vi "ArmPassThroughBodyWristAngle.vi"(0 "Arm Pass Through Params":T2, 1 "RobotDimensions":T1, 2 "PathIn":T3[](array[typedef])) -> (6 "PathOut":T3[](array[typedef]))   [LabVIEW 2018]
uses:
  TypeDefs/ArmCoordinate.ctl
  TypeDefs/ArmPassThroughParams.ctl
  TypeDefs/ConfigComponents/Config_Dimensions.ctl
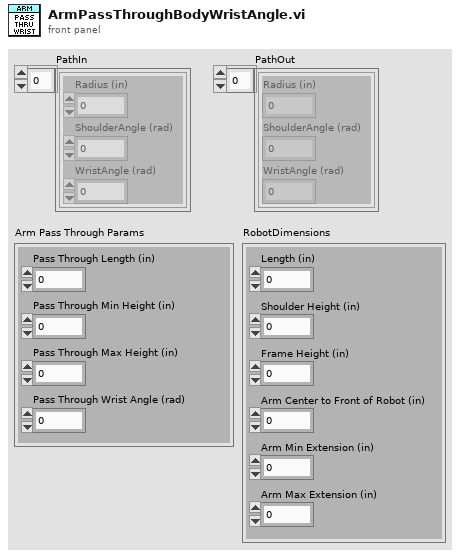
[diagram p1: front panel]
types:
  T1 = typedef "Config_Dimensions.ctl" = cluster{"Length (in)":dbl, "Shoulder Height (in)":dbl, "Frame Height (in)":dbl, "Arm Center to Front of Robot (in)":dbl, "Arm Min Extension (in)":dbl, "Arm Max Extension (in)":dbl}
  T2 = typedef "ArmPassThroughParams.ctl" = cluster{"Pass Through Length (in)":dbl, "Pass Through Min Height (in)":dbl, "Pass Through Max Height (in)":dbl, "Pass Through Wrist Angle (rad)":dbl}
  T3 = typedef "ArmCoordinate.ctl" = cluster{"Radius (in)":dbl, "ShoulderAngle (rad)":dbl, "WristAngle (rad)":dbl}
  T4 = typedef "ArmAbsolutePosition.ctl" = cluster{"X (in)":dbl, "Y (in)":dbl, "Wrist (rad)":dbl}
  T5 = typedef "ArgosLib.lvlib/Point2D.ctl" = cluster{"X (in)":dbl, "Y (in)":dbl}
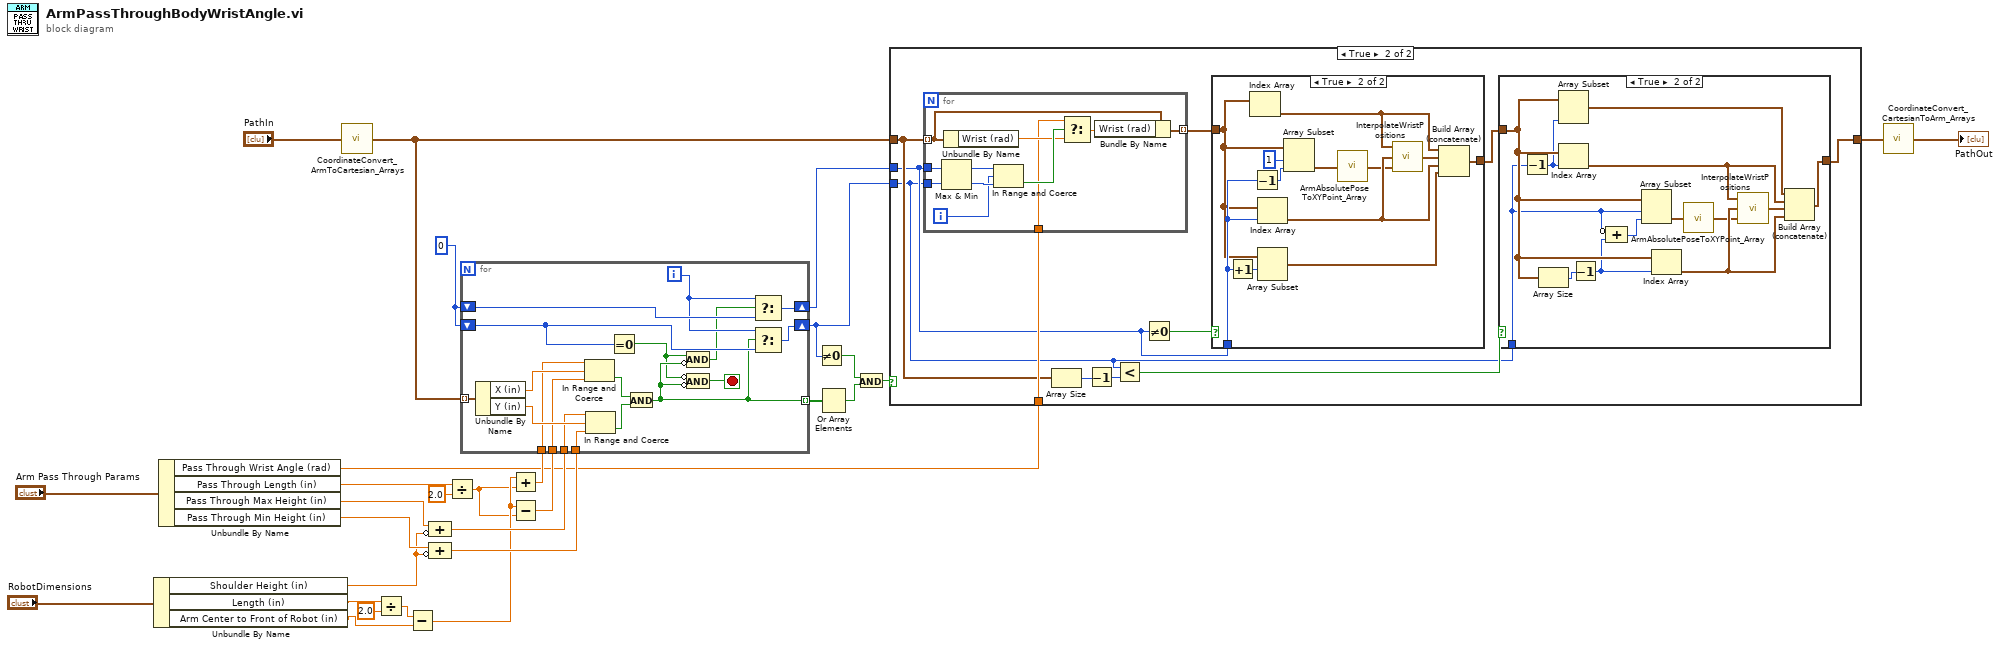
[diagram p0: block diagram]
diagram:
  w12 = 0
  n1 = Unbundle By Name("RobotDimensions") -> ("Shoulder Height (in)"=w21:dbl, "Length (in)"=w26:dbl, "Arm Center to Front of Robot (in)"=w24:dbl)
  n2 = Unbundle By Name("Arm Pass Through Params") -> ("Pass Through Wrist Angle (rad)"=w3:dbl, "Pass Through Length (in)"=w17:dbl, "Pass Through Max Height (in)"=w23:dbl, "Pass Through Min Height (in)"=w22:dbl)
  n3 = call "CoordinateConvert_ArmToCartesian_Arrays.vi"("ArmCoordinates"="PathIn") -> ("XYPoints"=w11:T4[])
  n4 = Divide(x=w26, y=2.0) -> (x/y=w25:dbl)
  n5 = Subtract(x=w25, y=w24) -> (x-y=w2:dbl)
  n6 = Compound Arithmetic op=ADD(w23, invert w21) -> (w14:dbl)
  n7 = Compound Arithmetic op=ADD(w22, invert w21) -> (w13:dbl)
  n8 = Divide(x=w17, y=2.0) -> (x/y=w1:dbl)
  n9 = Add(x=w2, y=w1) -> (x+y=w16:dbl)
  n10 = Subtract(x=w2, y=w1) -> (x-y=w15:dbl)
  n11 = for {
    tunnel: w11 -> [w47] mode=indexing
    tunnel: w16 -> [w44]
    tunnel: w15 -> [w43]
    tunnel: w14 -> [w42]
    tunnel: w13 -> [w41]
    tunnel: [w31] -> w10 mode=indexing
    shift-right: [w36] -> w4
    shift-left: w12 -> [w35]
    shift-right: [w38] -> w5
    shift-left: w12 -> [w37]
    i -> [w34]
    stop <- w32 stop-if-true
    n12 = Unbundle By Name(w47) -> ("X (in)"=w46:dbl, "Y (in)"=w45:dbl)
    n13 = In Range and Coerce(upper limit=w44, x=w46, lower limit=w43) -> (In Range?=w40:bool)  [unwired: 1 out]
    n14 = In Range and Coerce(upper limit=w42, x=w45, lower limit=w41) -> (In Range?=w39:bool)  [unwired: 1 out]
    n15 = Equal To 0?(x=w35) -> (x = 0?=w30:bool)
    n16 = And(x=w40, y=w39) -> (x .and. y?=w31:bool)
    n17 = Compound Arithmetic op=AND(w30, invert w31) -> (w33:bool)
    n18 = Compound Arithmetic op=AND(invert w30, invert w31) -> (w32:bool)
    n19 = Select(t=w34, s=w33, f=w37) -> (s? t:f=w38:i32)
    n20 = Select(t=w34, s=w31, f=w35) -> (s? t:f=w36:i32)
  }
  n21 = Not Equal To 0?(x=w4) -> (x != 0?=w9:bool)
  n22 = Or Array Elements(Boolean array=w10) -> (logical OR=w8:bool)
  n23 = And(x=w9, y=w8) -> (x .and. y?=w7:bool)
  n24 = case shown="True" w7 {
    tunnel: w11 -> [w48 w56]
    tunnel: [w48 w51] -> w6
    tunnel: w5 -> [_ w53]
    tunnel: w4 -> [_ w49]
    tunnel: w3 -> [_ w59]
    frame False {
    }
    frame True {
      n25 = for {
        tunnel: w53 -> [w97]
        tunnel: w49 -> [w96]
        tunnel: w56 -> [w92] mode=indexing
        tunnel: w59 -> [w88]
        tunnel: [w87] -> w57 mode=indexing
        i -> [w93]
        n26 = Max & Min(x=w97, y=w96) -> (max(x,y)=w95:i32, min(x,y)=w94:i32)
        n27 = Unbundle By Name(w92) -> ("Wrist (rad)"=w89:dbl)
        n28 = In Range and Coerce(upper limit=w95, x=w93, lower limit=w94) -> (In Range?=w90:bool)  [unwired: 1 out]
        n29 = Select(t=w88, s=w90, f=w89) -> (s? t:f=w91:dbl)
        n30 = Bundle By Name(cluster=w92, "Wrist (rad)"=w91) -> (w87:T4)
      }
      n31 = Array Size(array=w56) -> (size(s)=w55:i32)
      n32 = Decrement(x=w55) -> (x-1=w54:i32)
      n33 = Less?(x=w49, y=w54) -> (x < y?=w50:bool)
      n34 = Not Equal To 0?(x=w53) -> (x != 0?=w58:bool)
      n35 = case shown="True" w58 {
        tunnel: w57 -> [w74 w79]
        tunnel: [w74 w76] -> w52
        tunnel: w53 -> [_ w80]
        frame False {
        }
        frame True {
          n36 = Increment(x=w80) -> (x+1=w75:i32)
          n37 = Index Array(array=w79) -> (element=w86:T4)  [unwired: 1 in]
          n38 = Decrement(x=w80) -> (x-1=w81:i32)
          n39 = Index Array(array=w79, index=w80) -> (element=w85:T4)
          n40 = Array Subset(array=w79, index=w75) -> (w78:T4[])  [unwired: 1 in]
          n41 = Array Subset(array=w79, index=1, length=w81) -> (w82:T4[])
          n42 = call "ArmAbsolutePoseToXYPoint_Array.vi"("ArmAbsolutePose"=w82) -> ("2DPoint"=w77:T5[])
          n43 = call "InterpolateWristPositions.vi"("MiddlePoints"=w77, "SubsequentPose"=w85, "PriorPose"=w86) -> ("ConvertedPoints"=w84:T4[])
          n44 = Build Array (concatenate)(w86, w84, w85, w78) -> (w76:T4[])
        }
      }
      n45 = case shown="True" w50 {
        tunnel: w52 -> [w60 w66]
        tunnel: [w60 w68] -> w51
        tunnel: w49 -> [_ w61]
        frame False {
        }
        frame True {
          n46 = Decrement(x=w61) -> (x-1=w62:i32)
          n47 = Array Size(array=w66) -> (size(s)=w65:i32)
          n48 = Array Subset(array=w66, length=w62) -> (w67:T4[])  [unwired: 1 in]
          n49 = Index Array(array=w66, index=w62) -> (element=w73:T4)
          n50 = Decrement(x=w65) -> (x-1=w64:i32)
          n51 = Compound Arithmetic op=ADD(invert w61, w64) -> (w63:i32)
          n52 = Array Subset(array=w66, index=w61, length=w63) -> (w70:T4[])
          n53 = Index Array(array=w66, index=w64) -> (element=w72:T4)
          n54 = call "ArmAbsolutePoseToXYPoint_Array.vi"("ArmAbsolutePose"=w70) -> ("2DPoint"=w69:T5[])
          n55 = call "InterpolateWristPositions.vi"("MiddlePoints"=w69, "SubsequentPose"=w72, "PriorPose"=w73) -> ("ConvertedPoints"=w71:T4[])
          n56 = Build Array (concatenate)(w67, w73, w71, w72) -> (w68:T4[])
        }
      }
    }
  }
  n57 = call "CoordinateConvert_CartesianToArm_Arrays.vi"("XYPoints"=w6) -> ("ArmCoordinates"=→"PathOut":T3[])
